vi "Set-Frame-time.vi"(8 "error in (no error)":errorcluster, 9 "Frame rate":dbl caption="Frame rate [fps]", 10 "Frame time in":dbl caption="Frame time [s]", 11 "PF_MV1-D1312-240 in":refnum<class "PF_MV1-D1312-240.lvclass">) -> (0 "error out":errorcluster, 2 "Frame time":dbl caption="Frame time [s]", 3 "PF_MV1-D1312-240 out":refnum<class "PF_MV1-D1312-240.lvclass">)   [LabVIEW 2013, in "CameraVision.lvlib" / "PF_MV1-D1312-240.lvclass"]
uses:
  PF_MV1-D1312-240.lvclass
  Camera.lvclass/Camera.ctl
  <userlib>/Photonfocus Toolkit/_Public/SubVIs/pf_Set_Camera_Property_Float.vi
  <userlib>/Photonfocus Toolkit/_Public/SubVIs/pf_Set_Camera_Property_Bool.vi
  <userlib>/Photonfocus Toolkit/Photonfocus_Toolkit.lvlib
  Camera.lvclass
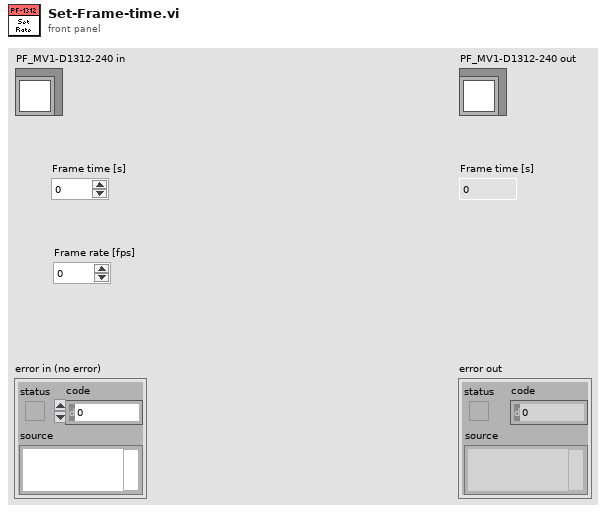
[diagram p1: front panel]
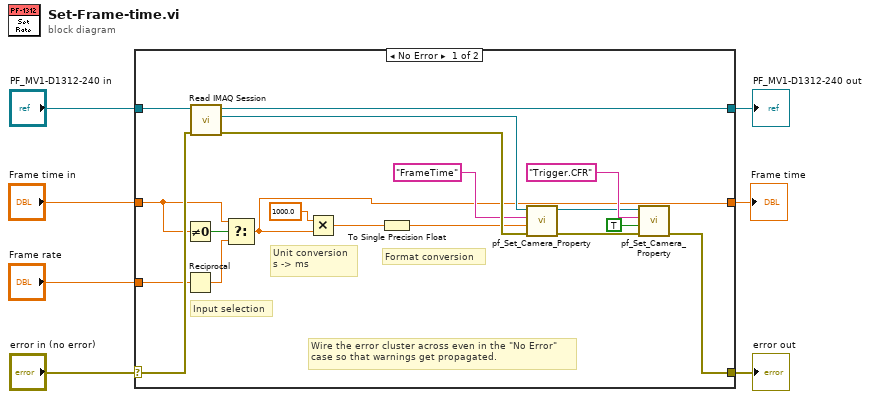
[diagram p0: block diagram]
diagram:
  n1 = case shown="No Error" "error in (no error)" {
    selector: "error in (no error)" -> [w23 w29]
    tunnel: [w12 w29] -> w6
    tunnel: [w24 w28] -> w4
    tunnel: "PF_MV1-D1312-240 in" -> [w25 w28]
    tunnel: "Frame time in" -> [w19 w27]
    tunnel: [w9 w27] -> w2
    tunnel: "Frame rate" -> [w10 _]
    frame No Error {
      # "Format conversion"
      # "Unit conversion\ns -> ms"
      # "Input selection"
      # "Wire the error cluster across even in the \"No Error\"\ncase so that warnings get propagated."
      n2 = Not Equal To 0?(x=w19) -> (x != 0?=w20:bool)
      n3 = Reciprocal(x=w10) -> (1/x=w11:dbl)
      n4 = call "Read IMAQ Session.vi"("error in (no error)"=w23, "Camera in"=w25) -> ("error out"=w22:errorcluster, "IMAQ Session"=w26:refnum<k11>, "Camera out"=w24:refnum<class "PF_MV1-D1312-240.lvclass">)  [unwired: 7 in]
      n5 = Select(t=w19, s=w20, f=w11) -> (s? t:f=w9:dbl)
      n6 = Multiply(x=1000.0, y=w9) -> (x*y=w18:dbl)
      n7 = To Single Precision Float(number=w18) -> (single precision float=w14:sgl)
      n8 = call-poly <userlib>:"pf_Set_Camera_Property.vi"("error in (no error)"=w22, "Property Value"=w14, "Property Name"="FrameTime", "IMAQ Session in"=w26) -> ("error out"=w16:errorcluster, "IMAQ Session out"=w13:refnum<k11>)  [unwired: 5 in, 1 out]
      n9 = call-poly <userlib>:"pf_Set_Camera_Property.vi"("error in (no error)"=w16, "Property Value"=TRUE, "Property Name"="Trigger.CFR", "IMAQ Session in"=w13) -> ("error out"=w12:errorcluster)  [unwired: 5 in, 2 out]
    }
    frame Error {
    }
  }
  "error out" <- w6
  "PF_MV1-D1312-240 out" <- w4
  "Frame time" <- w2
